vi "Test DIO.vi"() -> ()   [LabVIEW 2015]
uses:
  <vilib>/DAQmx/create/channels.llb/DAQmx Create Channel (CO-Pulse Generation-Frequency).vi
  <vilib>/DAQmx/configure/timing.llb/DAQmx Timing (Implicit).vi
panel:
  out "error out":errorcluster
  in  "Stop Button":bool
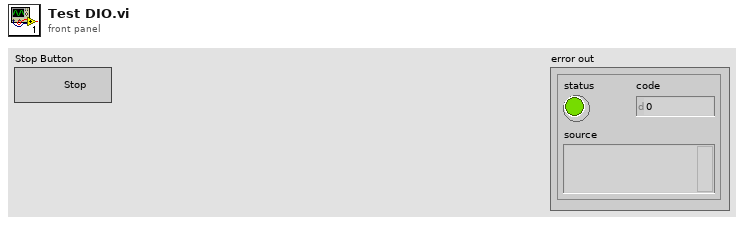
[diagram p1: front panel]
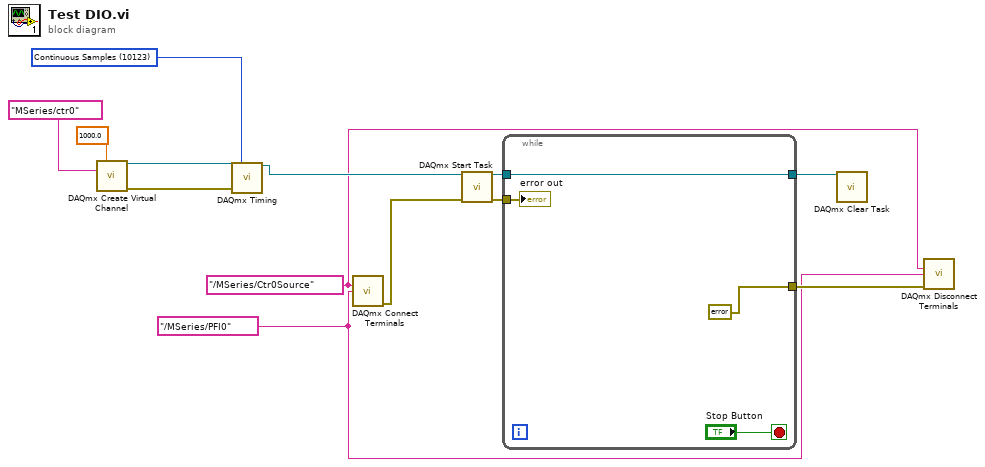
[diagram p0: block diagram]
diagram:
  w1 = tag "/MSeries/PFI0" ("destination terminal")
  w2 = tag "/MSeries/Ctr0Source" ("source terminal")
  w10 = 10123 items=["Finite Samples"=10178, "Continuous Samples"=10123, "Hardware Timed Single Point"=12522] ("sample mode")
  n1 = call-poly <vilib>:"DAQmx Create Virtual Channel.vi"("frequency"=1000.0, "counter"=tag "MSeries/ctr0") -> ("task out"=w12:refnum<k21>, "error out"=w11:errorcluster)  [unwired: 12 in]
  n2 = call-poly <vilib>:"DAQmx Timing.vi"("task/channels in"=w12, "sample mode"=w10, "error in"=w11) -> ("task out"=w9:refnum<k21>)  [unwired: 11 in, 1 out]
  n3 = call <vilib>:"DAQmx Connect Terminals.vi"("source terminal"=w2, "destination terminal"=w1) -> ("error out"=w4:errorcluster)  [unwired: 13 in]
  n4 = call <vilib>:"DAQmx Start Task.vi"("task/channels in"=w9, "error in"=w4) -> ("task out"=w7:refnum<k21>, "error out"=w8:errorcluster)  [unwired: 12 in]
  n5 = while {
    tunnel: w8 -> [w15]
    tunnel: w7 -> [w16]
    tunnel: [w16] -> w6
    tunnel: [errorcluster {"status"=FALSE, "code"=0, "source"=""} ("error out")] -> w3
    stop <- "Stop Button" stop-if-true
    "error out" <- w15
  }
  n6 = call <vilib>:"DAQmx Clear Task.vi"("task in"=w6) -> ()  [unwired: 14 in, 1 out]
  n7 = call <vilib>:"DAQmx Disconnect Terminals.vi"("source terminal"=w2, "destination terminal"=w1, "error in"=w3) -> ()  [unwired: 12 in, 1 out]
